vi "To File (Ref).vi"(6 "Pretty Print?":bool=TRUE, 7 "enable LabVIEW extensions? (T)":bool=TRUE, 8 "error in (no error)":errorcluster, 10 "JSON Value in":refnum<class "JSON Value.lvclass">, 11 "refnum in":refnum<file>) -> (0 "error out":errorcluster, 3 "refnum out":refnum<file>)   [LabVIEW 2016, in "JSON Value.lvclass"]
doc: "Saves a JSON instance's data to the given file."
uses:
  JSON Value.lvclass
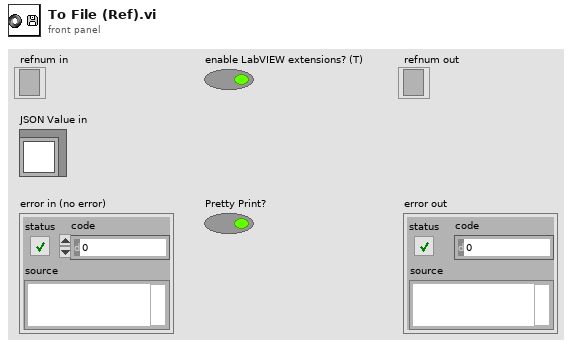
[diagram p1: front panel]
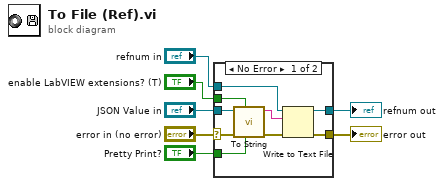
[diagram p0: block diagram]
diagram:
  n1 = case shown="No Error" "error in (no error)" {
    selector: "error in (no error)" -> [w14 w18]
    tunnel: "JSON Value in" -> [w16 _]
    tunnel: [w11 w18] -> w5
    tunnel: "Pretty Print?" -> [w9 _]
    tunnel: "refnum in" -> [w12 w17]
    tunnel: [w10 w17] -> w2
    tunnel: "enable LabVIEW extensions? (T)" -> [w8 _]
    frame No Error {
      n2 = call "To String.vi"("pretty print? (T)"=w9, "enable LabVIEW extensions? (T)"=w8, "error in (no error)"=w14, "JSON Value in"=w16) -> ("error out"=w13:errorcluster, "String"=w15:string)  [unwired: 6 in]
      n3 = Write to Text File(file (use dialog)=w12, text=w15, error in=w13) -> (refnum out=w10:refnum<file>, error out=w11:errorcluster)  [unwired: 1 in, 1 out]
    }
    frame Error {
    }
  }
  "error out" <- w5
  "refnum out" <- w2
